vi "Pwer_M test UI.vi"() -> ()   [LabVIEW 2021, in "Magnet module.lvlib" / "Power monitor.lvlib"]
uses:
  Power monitor.lvlib
  Messenger service/Data types/MSG to TOP.ctl
  Messenger service/Data types/Module name.ctl
  Typedefs/PwrM status.ctl
  .net PowerModeChanged/dotNET PowerModeChanged.llb/SystemPowerStatus.ctl
  Typedefs/PwrM commands.ctl
  Messenger service/MessengerLib.lvlib
panel:
  out "UPS out":T1 {"Last update" format="%<%H:%M:%S>T"}
  out "MSG packet":T2
  in  "force update":bool
  in  "stop":bool
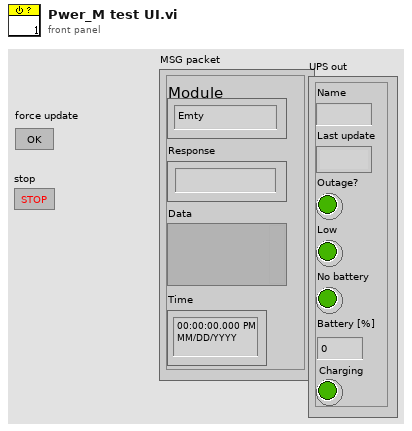
[diagram p1: front panel]
types:
  T1 = typedef "Magnet module.lvlib/Power monitor.lvlib/PwrM status.ctl" = cluster{"Name":string, "Last update":timestamp, "Outage?":bool, "Low":bool, "No battery":bool, "Battery [%]":u8, "Charging":bool}
  T2 = typedef "MessengerLib.lvlib/MSG to TOP.ctl" = cluster{"Module":T3, "Response":string, "Data":variant, "Time":timestamp}
  T3 = typedef "MessengerLib.lvlib/Module name.ctl" = enum16{"Emty", "Magnet", "VTI", "Excitation", "Servo", "Acquisition", "Rotator", "Digitizer", "SMU2450", "Carousel", "Multimeter", "Tmp monitor", "Power monitor"}
  T4 = typedef "SystemPowerStatus.ctl" = cluster{"ACLineStatus":u8, "BatteryFlag":u8, "BatteryLifePercent":u8, "Reserved":u8, "BatteryLifeTime":i32, "BatteryFullLifeTime":i32}
  T5 = typedef "Magnet module.lvlib/Power monitor.lvlib/PwrM commands.ctl" = enum16{"Ignore", "Update", "End"}
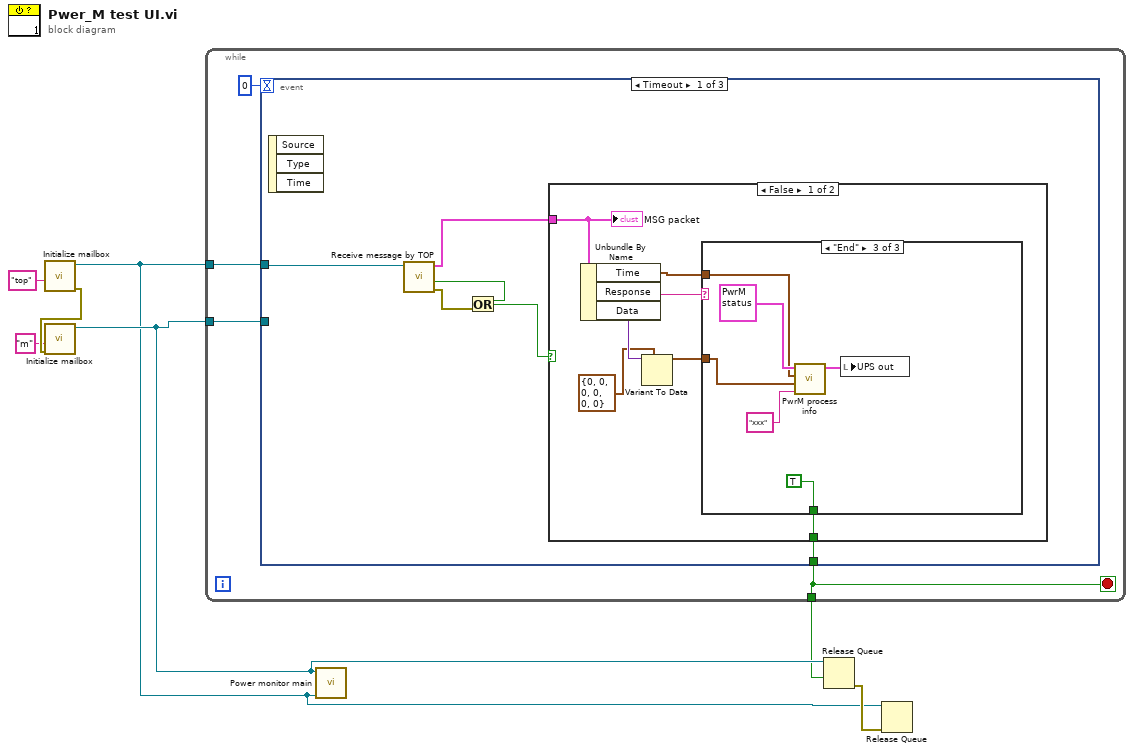
[diagram p0: block diagram]
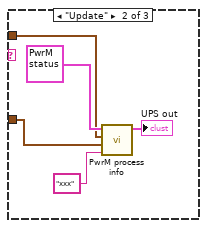
[diagram p3: hidden frame]
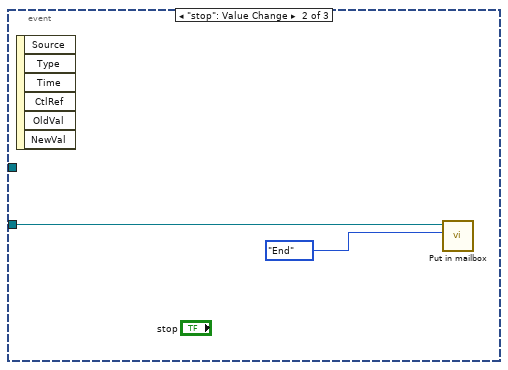
[diagram p5: hidden frame]
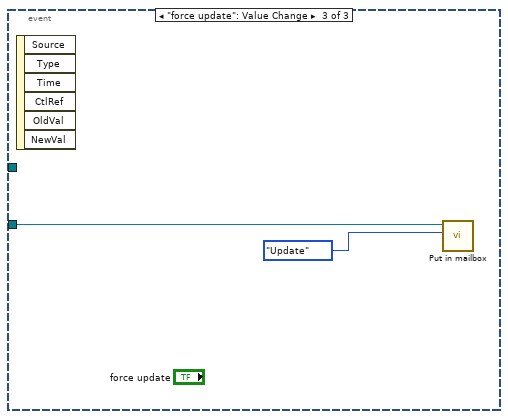
[diagram p6: hidden frame]
diagram:
  n1 = call "Initialize mailbox.vi"("name (unnamed)"="top") -> ("error out"=w7:errorcluster, "Queue out"=w2:refnum<queue>)  [unwired: 9 in]
  n2 = call "Initialize mailbox.vi"("error in"=w7, "name (unnamed)"="m") -> ("Queue out"=w4:refnum<queue>)  [unwired: 8 in, 1 out]
  n3 = while {
    tunnel: w2 -> [w11]
    tunnel: w4 -> [w10]
    tunnel: [w8] -> w1
    stop <- w8 stop-if-true
    n4 = event shown="[0] Timeout" {
      selector: _ -> [_ _ _]
      dyn-events: _ -> [_ _ _]
      timeout: 0 -> [_ _ _]
      tunnel: w11 -> [w17 _ _]
      tunnel: w10 -> [_ w37 w39]
      tunnel: [w12 _ _] -> w8
      event Timeout {
        n5 = event-data() -> ()  [unwired: 1 in, 3 out]
        n6 = call "Receive message by TOP.vi"("Mailbox in"=w17) -> ("error out"=w14:errorcluster, "timed out?"=w15:bool, "MSG packet"=w13:T2)  [unwired: 7 in, 1 out]
        n7 = Or(x=w15, y=w14) -> (x .or. y?=w16:bool)
        n8 = case shown="False" w16 {
          tunnel: w13 -> [w24 _]
          tunnel: [w18 _] -> w12
          frame False {
            n9 = Unbundle By Name(w24) -> ("Time"=w19:timestamp, "Response"=w22:string, "Data"=w23:variant)
            n10 = Variant To Data(type=T4 {"ACLineStatus"=0, "BatteryFlag"=0, "BatteryLifePercent"=0, "Reserved"=0, "BatteryLifeTime"=0, "BatteryFullLifeTime"=0} ("system_power_status"), Variant=w23) -> (data=w21:T4)  [unwired: 1 in, 1 out]
            n11 = case shown="\"End\"" w22 {
              tunnel: w21 -> [_ w28 w34]
              tunnel: w19 -> [_ w27 w33]
              tunnel: [_ _ TRUE] -> w18
              frame "Ignore", Default {
              }
              frame "Update" {
                n12 = call "PwrM process info.vi"("Name"="xxx", "PWR info cluster"=w28, "Timestamp"=w27, "UPS in"=T1 {"Name"="", "Last update"=timestamp(0 s since 1904-01-01), "Outage?"=FALSE, "Low"=FALSE, "No battery"=FALSE, "Battery [%]"=0, "Charging"=FALSE}) -> ("UPS out"=→"UPS out":T1)  [unwired: 7 in]
              }
              frame "End" {
                n13 = call "PwrM process info.vi"("Name"="xxx", "PWR info cluster"=w34, "Timestamp"=w33, "UPS in"=T1 {"Name"="", "Last update"=timestamp(0 s since 1904-01-01), "Outage?"=FALSE, "Low"=FALSE, "No battery"=FALSE, "Battery [%]"=0, "Charging"=FALSE}) -> ("UPS out"=w30:T1)  [unwired: 7 in]
                n14 = local write "UPS out"(w30) -> ()
              }
            }
            "MSG packet" <- w24
          }
          frame True {
          }
        }
      }
      event "stop": Value Change {
        n15 = event-data() -> ()  [unwired: 1 in, 6 out]
        n16 = call "Put in mailbox.vi"("Message"=PwrM_commands."End" ("Commands"), "Queue in"=w37) -> ()  [unwired: 7 in, 3 out]
      }
      event "force update": Value Change {
        n17 = event-data() -> ()  [unwired: 1 in, 6 out]
        n18 = call "Put in mailbox.vi"("Message"=PwrM_commands."Update" ("Commands"), "Queue in"=w39) -> ()  [unwired: 7 in, 3 out]
      }
    }
  }
  n19 = call "Power monitor main.vi"("Mailbox to TOP"=w2, "Module mailbox"=w4) -> ()  [unwired: 9 in, 1 out]
  n20 = Release Queue(queue=w4, force destroy? (F)=w1) -> (error out=w3:errorcluster)  [unwired: 1 in, 2 out]
  n21 = Release Queue(queue=w2, error in (no error)=w3) -> ()  [unwired: 1 in, 3 out]
